vi "DialogBox_twoButton_General_UIvi.vi"(6 "show close button?":bool, 7 "Boolean Text.Text":string, 8 "error in (no error)":errorcluster, 9 "Blink?":bool, 10 "Message Input":string, 11 "Dialog Box Input":string) -> (0 "error out":errorcluster, 3 "Proceed?":bool)   [LabVIEW 2015, in "ZenGage v3.0 UI.lvclass"]
uses:
  ZenGage v3.0 UI.lvclass
  Type Definitions/General/exit_General.ctl
panel:
  in  "error in (no error) 2":errorcluster
  in  "Clear":bool
  in  "cancel":T1
  out "Dialog Box out":string
  in  "OK button":bool
  out "Message":string
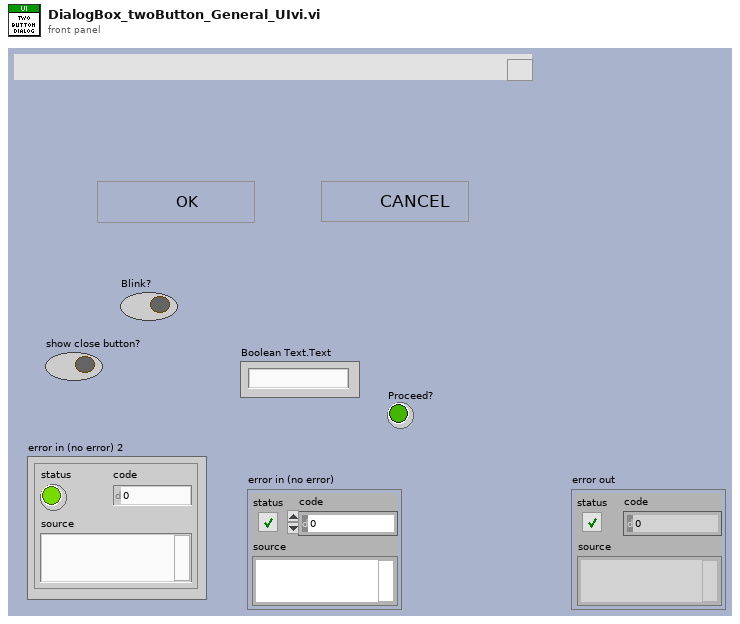
[diagram p1: front panel]
types:
  T1 = typedef "ZenGage v3.0 UI.lvclass/exit_General.ctl" = bool
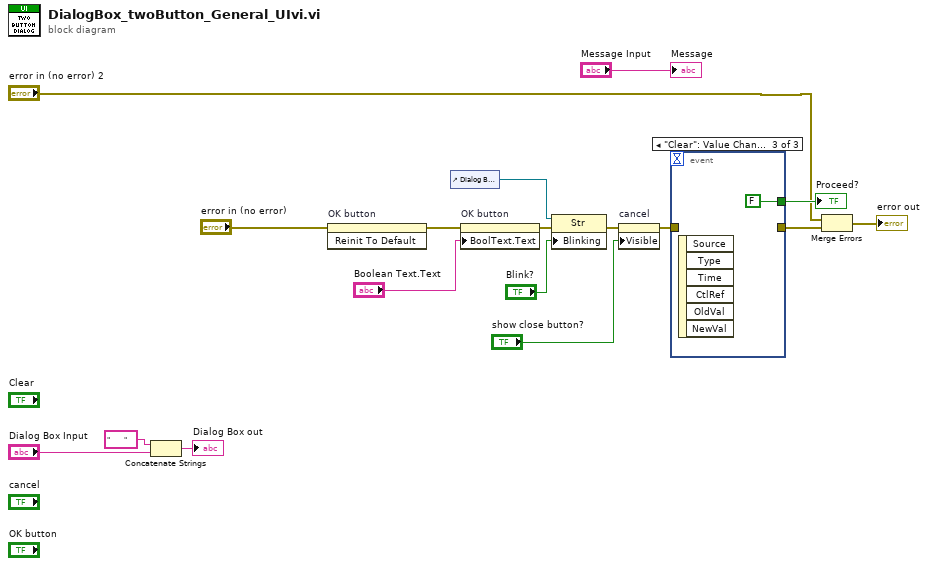
[diagram p0: block diagram]
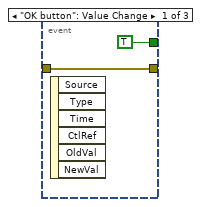
[diagram p2: hidden frame]
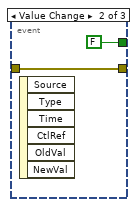
[diagram p3: hidden frame]
diagram:
  n1 = Concatenate Strings("       " ("string"), "Dialog Box Input") -> (→"Dialog Box out":string)
  n2 = invoke on="OK button" class="Bool (strict)" method="Reinit To Default"(error in="error in (no error)") -> (error out=w7:errorcluster)  [unwired: 2 in, 2 out]
  n3 = control-ref of="Dialog Box out"() -> (w15:refnum<vi>)
  n4 = property on="OK button" class="Bool (strict)"(error in=w7, "BoolText.Text"="Boolean Text.Text") -> (error out=w6:errorcluster)  [unwired: 1 in, 1 out]
  n5 = property class="Str"(reference=w15, error in=w6, "Blinking"="Blink?") -> (error out=w11:errorcluster)  [unwired: 1 out]
  n6 = property on="cancel" class="Bool"(error in=w11, "Visible"="show close button?") -> (error out=w10:errorcluster)  [unwired: 1 in, 1 out]
  n7 = event shown="[2] \"Clear\": Value Change" {
    selector: _ -> [_ _ _]
    dyn-events: _ -> [_ _ _]
    timeout: _ -> [_ _ _]
    tunnel: [TRUE FALSE FALSE] -> w17
    tunnel: w10 -> [w18 w20 _]
    tunnel: [w18 w20 _] -> w4
    event "OK button": Value Change {
      n8 = event-data() -> ()  [unwired: 1 in, 6 out]
    }
    event Value Change {
      n9 = event-data() -> ()  [unwired: 1 in, 6 out]
    }
    event "Clear": Value Change {
      n10 = event-data() -> ()  [unwired: 1 in, 6 out]
    }
  }
  "Proceed?" <- w17
  n11 = Merge Errors("error in (no error) 2", w4) -> (→"error out":errorcluster)
  "Message" <- "Message Input"
